vi "Global 1.vi"() -> ()   [LabVIEW 2014]
panel:
  in  "Stop Saving":bool
  in  "Start Saving":bool
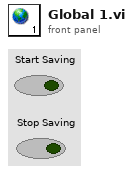
[diagram p1: front panel]
diagram:
